vi "Do Action.vi"(0 "Serial port asssistant model in":refnum<class "Serial port assistant model.lvclass">, 7 "request":string, 11 "error in (no error)":errorcluster) -> (4 "Serial port asssistant model out":refnum<class "Serial port assistant model.lvclass">, 15 "error out":errorcluster)   [LabVIEW 2022 SP3, in "Serial port assistant model.lvlib" / "Serial port assistant model.lvclass"]
uses:
  Serial port assistant model.lvclass
  <vilib>/Instr/_visa.llb/VISA Find Search Mode.ctl
  Serial port assistant model.lvclass/Serial port assistant model.ctl
  <vilib>/Instr/_visa.llb/VISA Configure Serial Port (Instr).vi
  receive data.vi
panel:
  in  "stop receiving data":bool
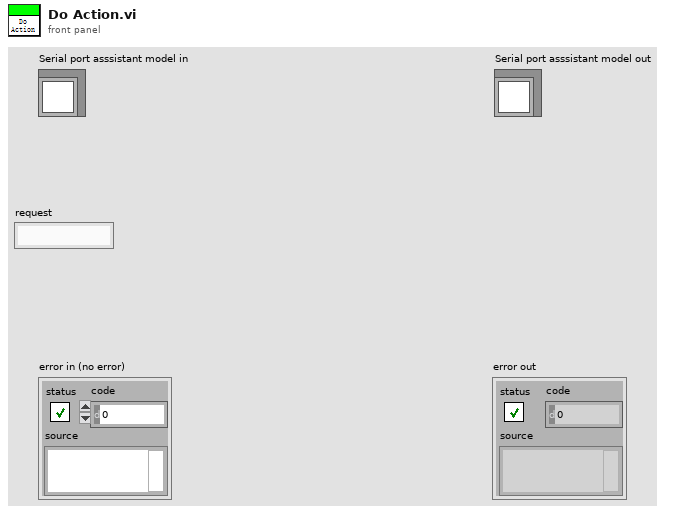
[diagram p1: front panel]
types:
  T1 = cluster{"changed data":string, "serial port list":string[]}
  T2 = cluster{"serial port":string, "baud rate":u32, "data bits":u16, "stop bits":u16, "parity":u16}
  T3 = cluster{"changed data":string, "serial port":string, "baud rate":u32, "data bits":u16, "stop bits":u16, "parity":u16, "open":bool}
  T4 = cluster{"changed data":string, "send time":string, "data has been sent":string}
  T5 = typedef "VISA Find Search Mode.ctl" = u32
  T6 = typedef "Rendezvous RefNum" = refnum<k1>
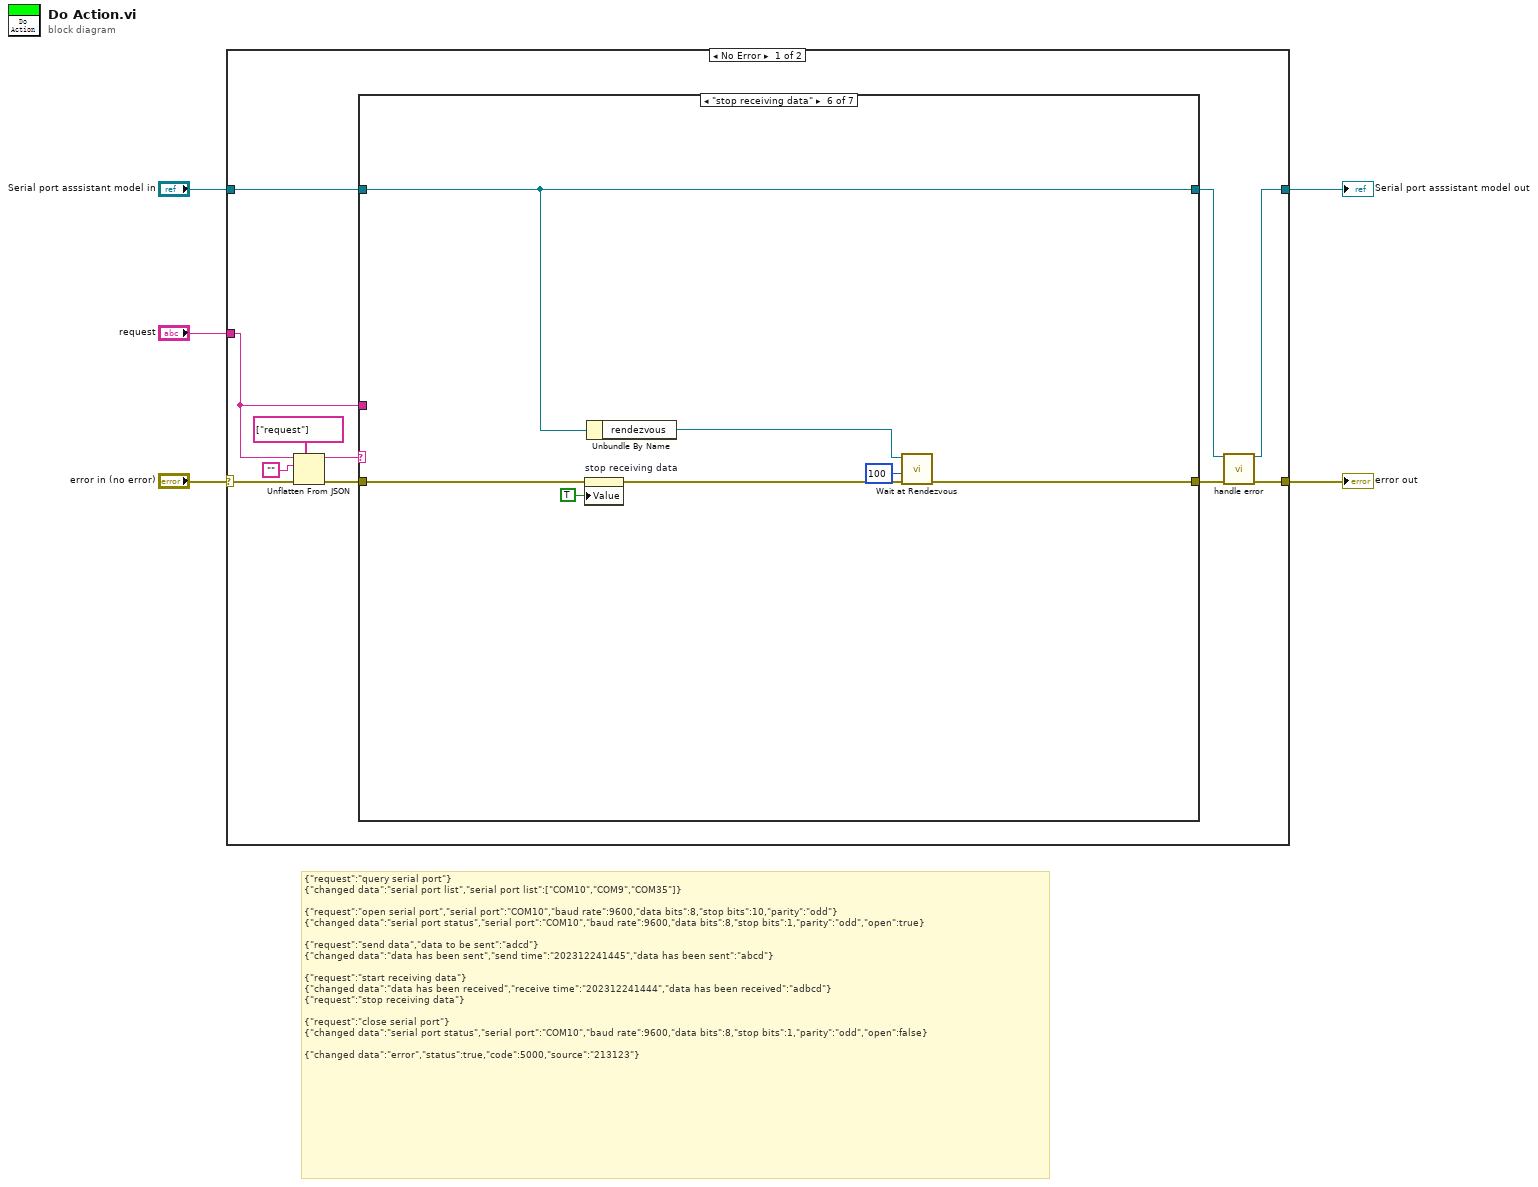
[diagram p0: block diagram]
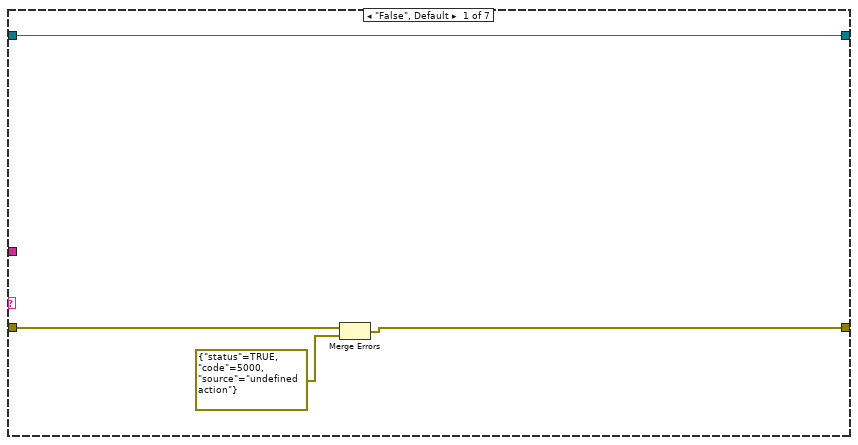
[diagram p2: hidden frame]
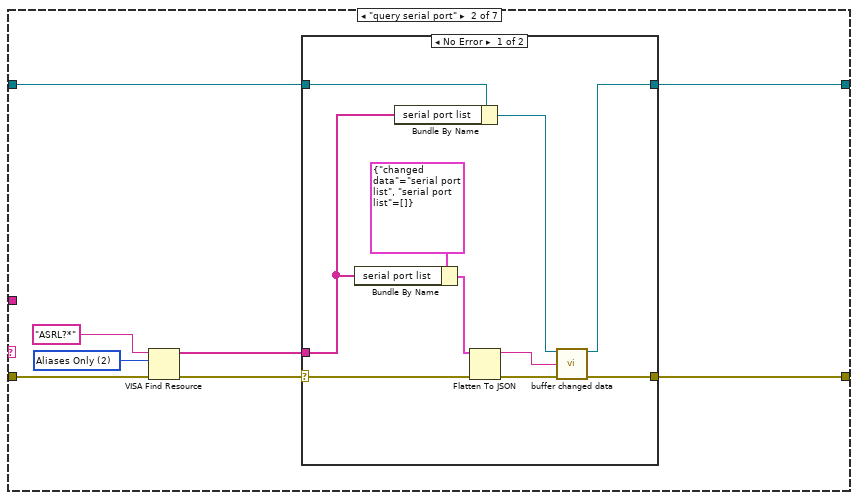
[diagram p3: hidden frame]
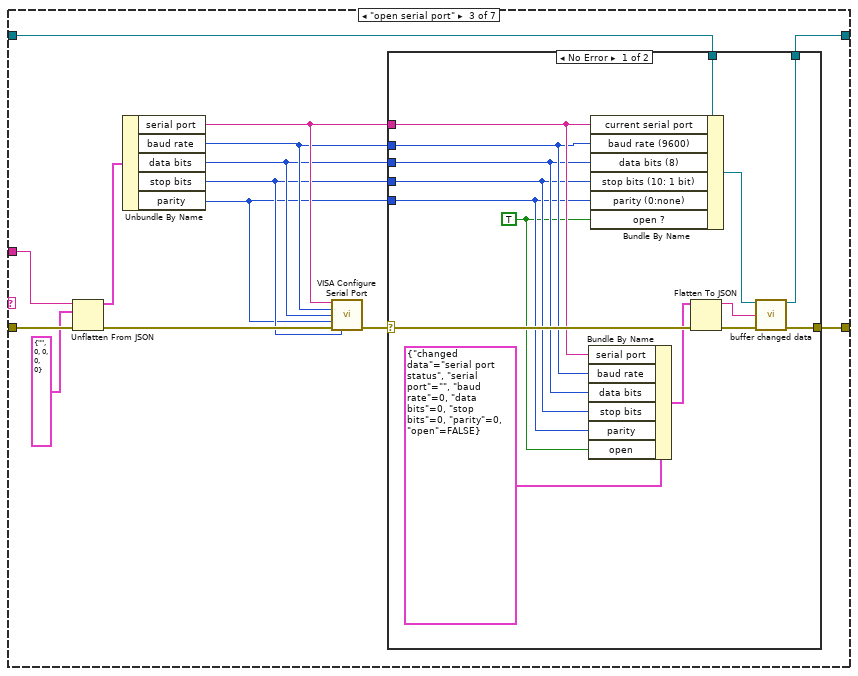
[diagram p5: hidden frame]
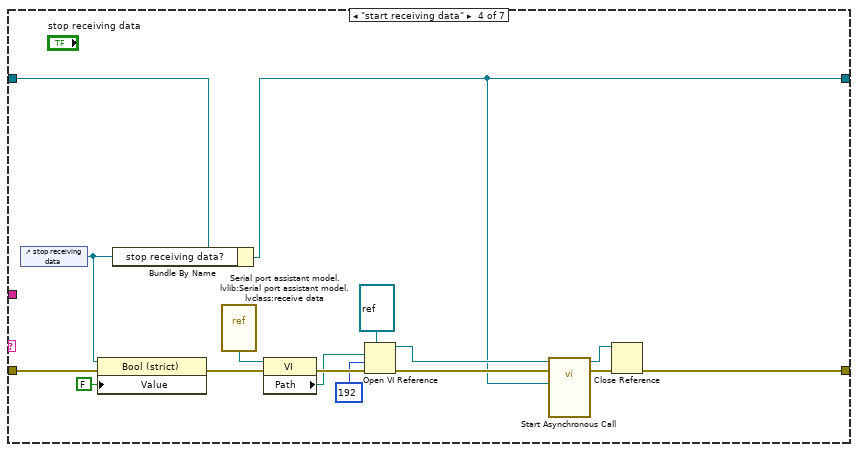
[diagram p7: hidden frame]
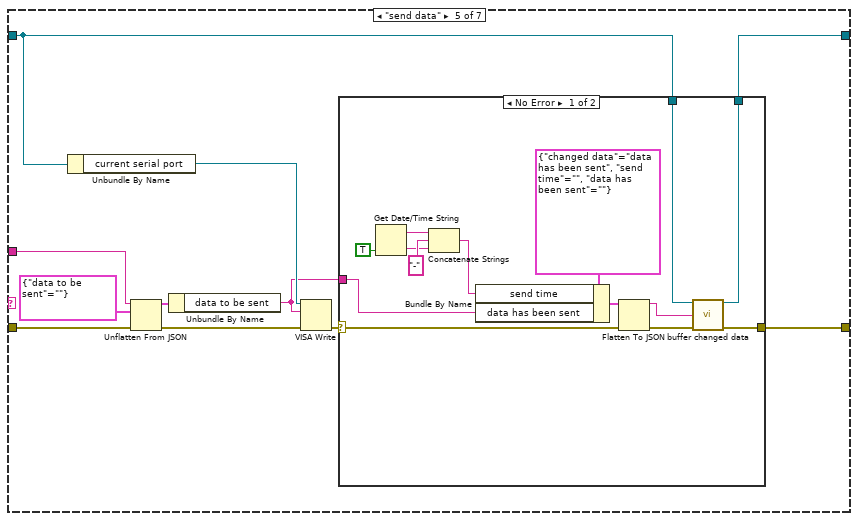
[diagram p8: hidden frame]
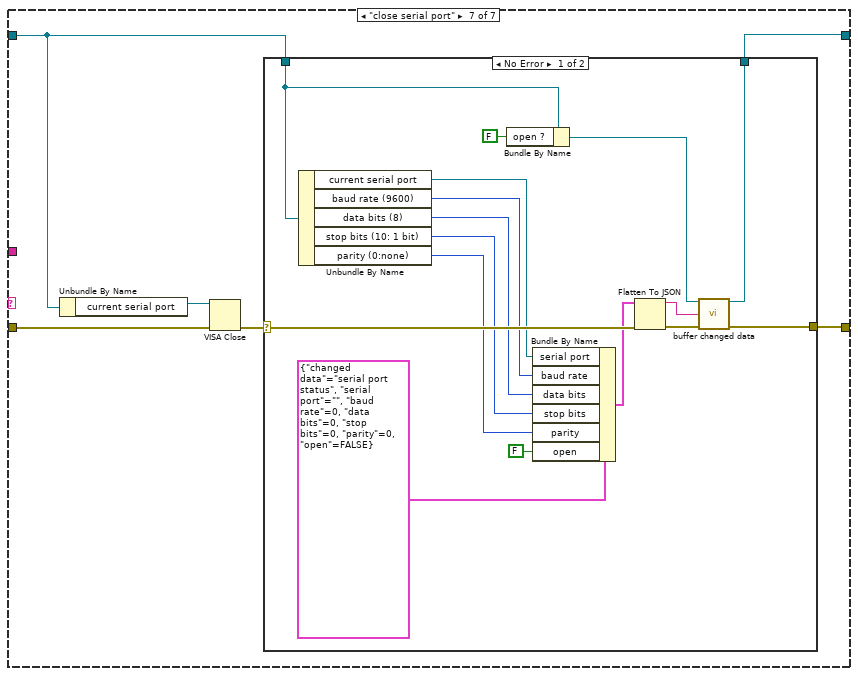
[diagram p10: hidden frame]
diagram:
  # "{\"request\":\"query serial port\"}         \n{\"changed data\":\"serial port list\",\"serial port list\":[\"COM10\",\"COM9\",\"COM35\"]}\n\n{\"request\":\"open serial port\",\"serial port\":\"COM10\",\"baud rate\":9600,\"data bits\":8,\"stop bits\":10,\"parity\":\"odd\"}       \n{\"changed data\":\"serial port status\",\"serial port\":\"COM10\",\"baud rate\":9600,\"data bits\":8,\"stop bits\":1,\"parity\":\"odd\",\"open\":true}\n\n{\"request\":\"send data\",\"data to be sent\":\"adcd\"}                 \n{\"changed data\":\"data has been sent\",\"send time\":\"202312241445\",\"data has been sent\":\"abcd\"}\n\n{\"request\":\"start receiving data\"}\n{\"changed data\":\"data has been received\",\"receive time\":\"202312241444\",\"data has been received\":\"adbcd\"}\n{\"request\":\"stop receiving data\"}\n\n{\"request\":\"close serial port\"}          \n{\"changed data\":\"serial port status\",\"serial port\":\"COM10\",\"baud rate\":9600,\"data bits\":8,\"stop bits\":1,\"parity\":\"odd\",\"open\":false}\n\n{\"changed data\":\"error\",\"status\":true,\"code\":5000,\"source\":\"213123\"}"
  n1 = case shown="No Error" "error in (no error)" {
    selector: "error in (no error)" -> [w14 w146]
    tunnel: [w8 w146] -> w1
    tunnel: "Serial port asssistant model in" -> [w11 w147]
    tunnel: [w6 w147] -> w2
    tunnel: "request" -> [w10 _]
    frame No Error {
      n2 = Unflatten From JSON(path=string[] ["request"], JSON string=w10, type and defaults="", error in (no error)=w14) -> (value=w13:string, error out=w12:errorcluster)  [unwired: 3 in]
      n3 = case shown="\"stop receiving data\"" w13 {
        tunnel: w12 -> [w19 w26 w54 w73 w98 w121 w127]
        tunnel: w11 -> [w18 w24 w52 w77 w88 w119 w124]
        tunnel: [w18 w23 w45 w76 w89 w119 w123] -> w7
        tunnel: [w17 w21 w48 w78 w90 w117 w122] -> w9
        tunnel: w10 -> [_ _ w53 _ w94 _ _]
        frame "False", Default {
          n4 = Merge Errors(w19, errorcluster {"status"=TRUE, "code"=5000, "source"="undefined action"} ("error out")) -> (w17:errorcluster)
        }
        frame "query serial port" {
          w28 = T5 2 items=["Canonical Names Only"=0, "Aliases Only"=2, "Include Matching Aliases"=3, "Include All Aliases"=4] ("Search Mode")
          n5 = VISA Find Resource(8:w26, 10:w28, 11:"ASRL?*" ("expression (\"?*\")")) -> (0:w25:errorcluster, 3:w22:string[])  [unwired: 1 out]
          n6 = case shown="No Error" w25 {
            selector: w25 -> [w35 w39]
            tunnel: w24 -> [w38 w40]
            tunnel: [w31 w40] -> w23
            tunnel: w22 -> [w29 _]
            tunnel: [w33 w39] -> w21
            frame No Error {
              n7 = Bundle By Name(cluster=T1 {"changed data"="serial port list", "serial port list"=[]}, "serial port list"=w29) -> (w36:T1)
              n8 = Bundle By Name(cluster=w38, "serial port list"=w29) -> (w32:refnum<class "Serial port assistant model.lvclass">)
              n9 = Flatten To JSON(anything=w36, error in (no error)=w35) -> (JSON string=w30:string, 11:w34:errorcluster)  [unwired: 1 in]
              n10 = call "buffer changed data.vi"("Serial port asssistant model in"=w32, "changed data"=w30, "error in (no error)"=w34) -> ("Serial port asssistant model out"=w31:refnum<class "Serial port assistant model.lvclass">, "error out"=w33:errorcluster)  [unwired: 11 in]
            }
            frame Error {
            }
          }
        }
        frame "open serial port" {
          n11 = Unflatten From JSON(JSON string=w53, type and defaults=T2 {"serial port"="", "baud rate"=0, "data bits"=0, "stop bits"=0, "parity"=0} ("serial port status"), error in (no error)=w54) -> (value=w50:T2, error out=w51:errorcluster)  [unwired: 4 in]
          n12 = Unbundle By Name(w50) -> ("serial port"=w47:string, "baud rate"=w46:u32, "data bits"=w44:u16, "stop bits"=w43:u16, "parity"=w41:u16)
          n13 = call-poly "VISA Configure Serial Port"("VISA resource name"=w47, "baud rate (9600)"=w46, "data bits (8)"=w44, "parity (0:none)"=w41, "error in (no error)"=w51, "stop bits (10: 1 bit)"=w43) -> ("error out"=w49:errorcluster)  [unwired: 8 in, 1 out]
          n14 = case shown="No Error" w49 {
            selector: w49 -> [w67 w71]
            tunnel: w52 -> [w69 w70]
            tunnel: [w66 w71] -> w48
            tunnel: w47 -> [w64 _]
            tunnel: w46 -> [w63 _]
            tunnel: [w55 w70] -> w45
            tunnel: w44 -> [w62 _]
            tunnel: w43 -> [w61 _]
            tunnel: w41 -> [w60 _]
            frame No Error {
              w59 = TRUE ("open ?")
              n15 = Bundle By Name(cluster=T3 {"changed data"="serial port status", "serial port"="", "baud rate"=0, "data bits"=0, "stop bits"=0, "parity"=0, "open"=FALSE} ("serial port status"), "serial port"=w64, "baud rate"=w63, "data bits"=w62, "stop bits"=w61, "parity"=w60, "open"=w59) -> (w58:T3)
              n16 = Bundle By Name(cluster=w69, "current serial port"=w64, "baud rate (9600)"=w63, "data bits (8)"=w62, "stop bits (10: 1 bit)"=w61, "parity (0:none)"=w60, "open ?"=w59) -> (w56:refnum<class "Serial port assistant model.lvclass">)
              n17 = Flatten To JSON(anything=w58, error in (no error)=w67) -> (JSON string=w57:string, 11:w68:errorcluster)  [unwired: 1 in]
              n18 = call "buffer changed data.vi"("Serial port asssistant model in"=w56, "changed data"=w57, "error in (no error)"=w68) -> ("Serial port asssistant model out"=w55:refnum<class "Serial port assistant model.lvclass">, "error out"=w66:errorcluster)  [unwired: 11 in]
            }
            frame Error {
            }
          }
        }
        frame "start receiving data" {
          n19 = control-ref of="stop receiving data"() -> (w75:refnum<vi>)
          n20 = property class="Bool (strict)"(reference=w75, error in=w73, "Value"=FALSE) -> (error out=w72:errorcluster)  [unwired: 1 out]
          n21 = Bundle By Name(cluster=w77, "stop receiving data?"=w75) -> (w76:refnum<class "Serial port assistant model.lvclass">)
          n22 = vi-ref "Serial port assistant model.lvlib:Serial port assistant model.lvclass:receive data.vi"() -> (w87:refnum<vi>)
          n23 = property class="VI"(reference=w87, error in=w72) -> (error out=w85:errorcluster, "Path"=w84:path)  [unwired: 1 out]
          n24 = Open VI Reference(type specifier VI Refnum (for type only)=refnum<vi> refnum, vi path=w84, options=192, error in (no error)=w85) -> (vi reference=w82:refnum<vi>, error out=w81:errorcluster)  [unwired: 2 in]
          n25 = call-by-ref "Start Asynchronous Call"(reference=w82, error in=w81, "Serial port asssistant model in"=w76) -> (reference out=w79:refnum<vi>, error out=w80:errorcluster)  [unwired: 14 in, 1 out]
          n26 = Close Reference(reference=w79, error in (no error)=w80) -> (error out=w78:errorcluster)
        }
        frame "send data" {
          n27 = Unbundle By Name(w88) -> ("current serial port"=w96:refnum<visa-resource-name>)
          n28 = Unflatten From JSON(JSON string=w94, type and defaults=cluster{"data to be sent":string} {"data to be sent"=""}, error in (no error)=w98) -> (value=w93:cluster{"data to be sent":string}, error out=w97:errorcluster)  [unwired: 4 in]
          n29 = Unbundle By Name(w93) -> ("data to be sent"=w91:string)
          n30 = VISA Write(VISA resource name=w96, write buffer=w91, error in (no error)=w97) -> (error out=w92:errorcluster)  [unwired: 2 out]
          n31 = case shown="No Error" w92 {
            selector: w92 -> [w112 w113]
            tunnel: w91 -> [w101 _]
            tunnel: [w110 w113] -> w90
            tunnel: w88 -> [w108 w114]
            tunnel: [w107 w114] -> w89
            frame No Error {
              n32 = Get Date/Time String(want seconds? (F)=TRUE) -> (date string=w105:string, time string=w103:string)  [unwired: 2 in]
              n33 = Concatenate Strings(w105, "-" ("string"), w103) -> (w99:string)
              n34 = Bundle By Name(cluster=T4 {"changed data"="data has been sent", "send time"="", "data has been sent"=""}, "send time"=w99, "data has been sent"=w101) -> (w100:T4)
              n35 = Flatten To JSON(anything=w100, error in (no error)=w112) -> (JSON string=w109:string, 11:w111:errorcluster)  [unwired: 1 in]
              n36 = call "buffer changed data.vi"("Serial port asssistant model in"=w108, "changed data"=w109, "error in (no error)"=w111) -> ("Serial port asssistant model out"=w107:refnum<class "Serial port assistant model.lvclass">, "error out"=w110:errorcluster)  [unwired: 11 in]
            }
            frame Error {
            }
          }
        }
        frame "stop receiving data" {
          n37 = property on="stop receiving data" class="Bool (strict)"(error in=w121, "Value"=TRUE ("stop receiving data")) -> (error out=w118:errorcluster)  [unwired: 1 in, 1 out]
          n38 = Unbundle By Name(w119) -> ("rendezvous"=w116:T6)
          n39 = call <vilib>:"Wait at Rendezvous.vi"("error in (no error)"=w118, "ms timeout (-1)"=100, "rendezvous"=w116) -> ("error out"=w117:errorcluster)  [unwired: 2 in, 2 out]
        }
        frame "close serial port" {
          n40 = Unbundle By Name(w124) -> ("current serial port"=w126:refnum<visa-resource-name>)
          n41 = VISA Close(VISA resource name=w126, error in (no error)=w127) -> (error out=w125:errorcluster)
          n42 = case shown="No Error" w125 {
            selector: w125 -> [w141 w144]
            tunnel: w124 -> [w140 w145]
            tunnel: [w129 w145] -> w123
            tunnel: [w128 w144] -> w122
            frame No Error {
              n43 = Unbundle By Name(w140) -> ("current serial port"=w137:refnum<visa-resource-name>, "baud rate (9600)"=w136:u32, "data bits (8)"=w135:u16, "stop bits (10: 1 bit)"=w134:u16, "parity (0:none)"=w133:enum16{"None", "Odd", "Even", "Mark", "Space"})
              n44 = Bundle By Name(cluster=w140, "open ?"=FALSE) -> (w130:refnum<class "Serial port assistant model.lvclass">)
              n45 = Bundle By Name(cluster=T3 {"changed data"="serial port status", "serial port"="", "baud rate"=0, "data bits"=0, "stop bits"=0, "parity"=0, "open"=FALSE} ("serial port status"), "serial port"=w137, "baud rate"=w136, "data bits"=w135, "stop bits"=w134, "parity"=w133, "open"=FALSE) -> (w131:T3)
              n46 = Flatten To JSON(anything=w131, error in (no error)=w141) -> (JSON string=w142:string, 11:w143:errorcluster)  [unwired: 1 in]
              n47 = call "buffer changed data.vi"("Serial port asssistant model in"=w130, "changed data"=w142, "error in (no error)"=w143) -> ("Serial port asssistant model out"=w129:refnum<class "Serial port assistant model.lvclass">, "error out"=w128:errorcluster)  [unwired: 11 in]
            }
            frame Error {
            }
          }
        }
      }
      n48 = call "handle error.vi"("Serial port assistant model in"=w7, "error in (no error)"=w9) -> ("Serial port assistant model out"=w6:refnum<class "Serial port assistant model.lvclass">, "error out"=w8:errorcluster)  [unwired: 12 in]
    }
    frame Error {
    }
  }
  "error out" <- w1
  "Serial port asssistant model out" <- w2
